vi "Custom User Scripting For New Override VI.vi"(8 "error in":errorcluster, 11 "VI Refnum in":refnum<vi>) -> (0 "error out":errorcluster)   [LabVIEW 2012]
doc: "When \"New >> VI For Override...\" is used to create a VI, this subVI will be invoked if the VI is created successfully after all other work to create the VI has been completed. Users may edit this subVI to add any instructions they wish for customizations of the newly generated VI."
uses:
  <vilib>/regexp/Match Regular Expression.xnode
  <vilib>/Utility/miscctls.llb/LVRectTypeDef.ctl
panel:
  out "error out 2":errorcluster
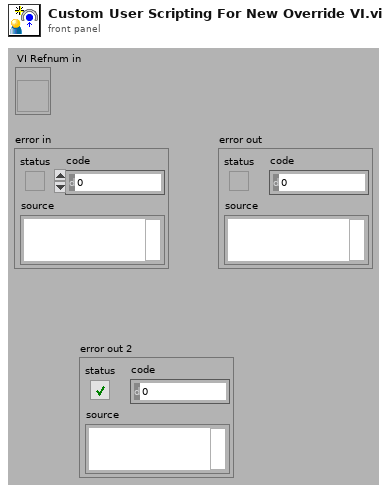
[diagram p1: front panel]
types:
  T1 = typedef "LVRectTypeDef.ctl" = cluster{"Left":i16, "Top":i16, "Right":i16, "Bottom":i16}
  T2 = cluster{"Class In":refnum<vi>, "Class Out":refnum<vi>, "Error In":refnum<vi>, "Error Out":refnum<vi>, "Other In":refnum<vi>[], "Other Out":refnum<vi>[]}
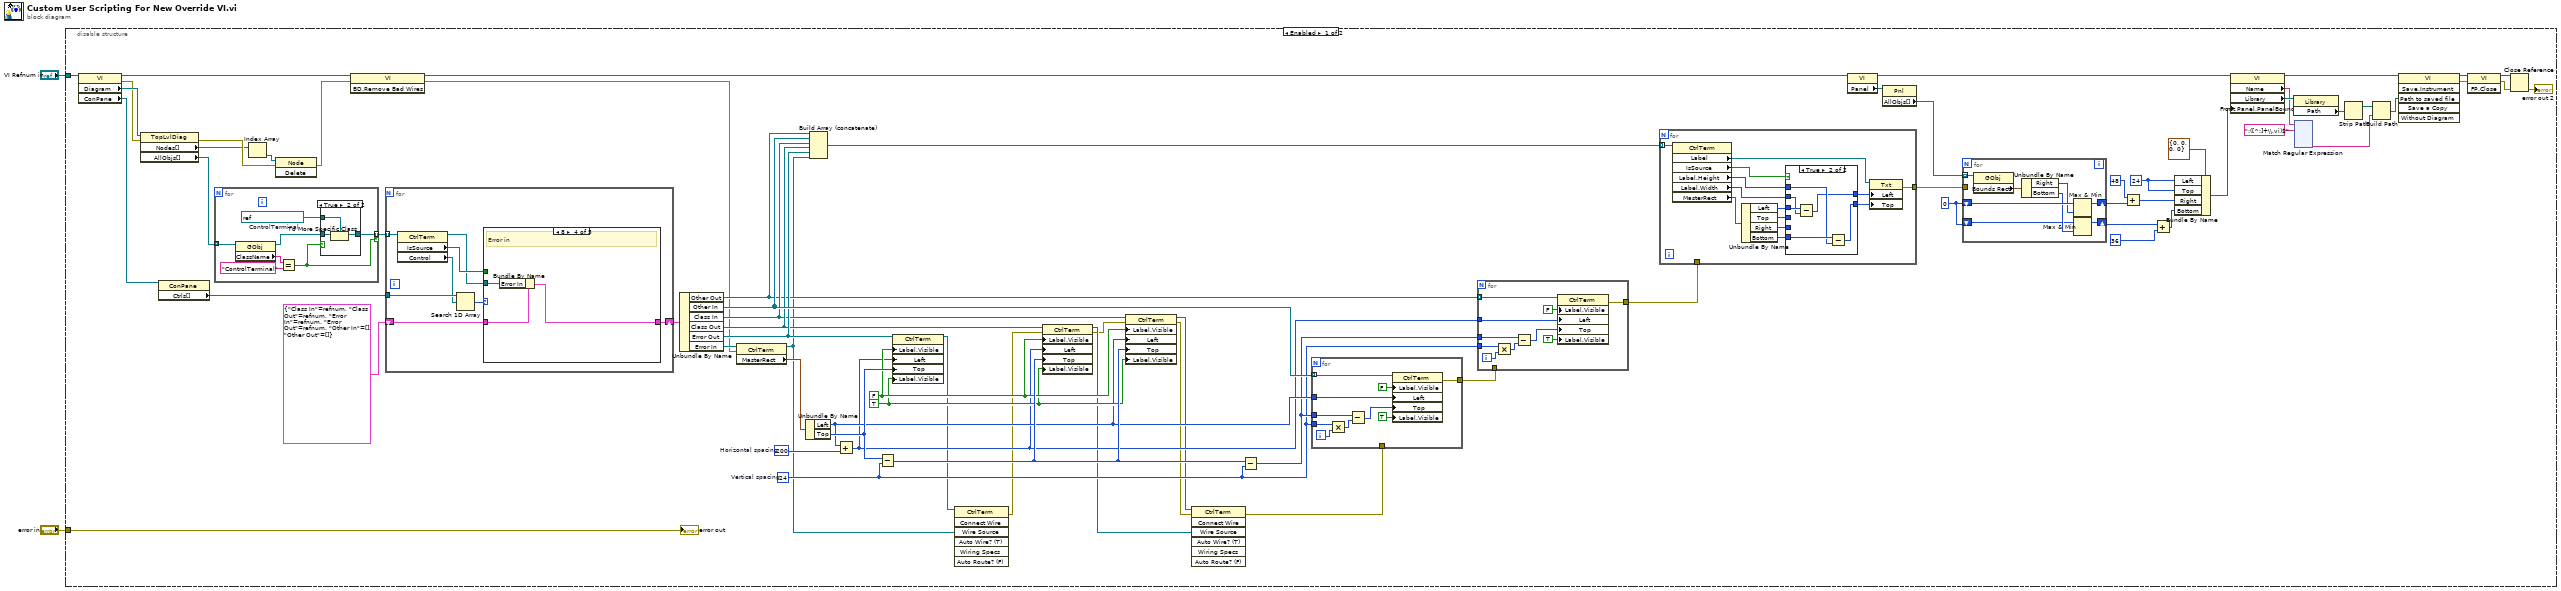
[diagram p0: block diagram]
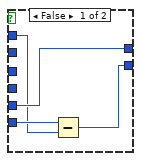
[diagram p2: hidden frame]
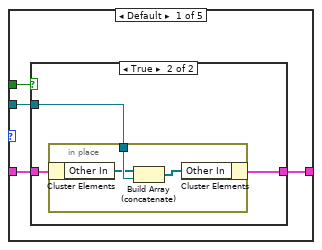
[diagram p3: hidden frame]
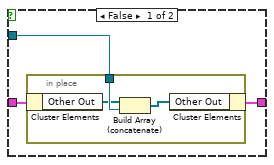
[diagram p4: hidden frame]
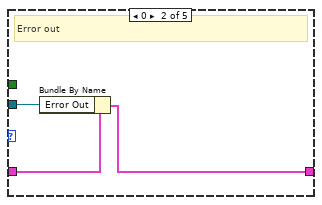
[diagram p5: hidden frame]
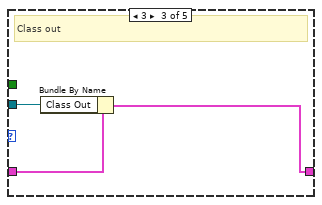
[diagram p6: hidden frame]
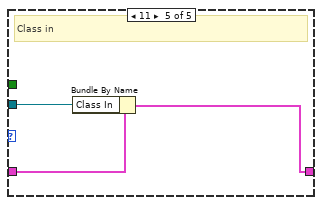
[diagram p7: hidden frame]
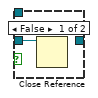
[diagram p8: hidden frame]
diagram:
  n1 = disable-structure shown="Enabled" {
    disable-tunnel: "error in" -> [w71 _]
    disable-tunnel: "VI Refnum in" -> [w70 _]
    frame Enabled {
      w13 = i16 24 ("x")
      w21 = i16 0 ("Right")
      w50 = TRUE ("Label.Visible")
      w51 = FALSE ("Label.Visible")
      w45 = 24  # Vertical spacing
      w61 = 200  # Horizontal spacing
      n2 = property class="VI"(reference=w70) -> (reference out=w24:refnum<vi>, error out=w66:errorcluster, "Diagram"=w69:refnum<vi>, "ConPane"=w39:refnum<vi>)  [unwired: 1 in]
      n3 = property class="TopLvlDiag"(reference=w69, error in=w66) -> (error out=w72:errorcluster, "Nodes[]"=w68:refnum<vi>[], "AllObjs[]"=w40:refnum<vi>[])  [unwired: 1 out]
      n4 = property class="ConPane"(reference=w39) -> ("Ctrls[]"=w64:refnum<vi>[])  [unwired: 1 in, 2 out]
      n5 = for {
        tunnel: w40 -> [w156] mode=indexing
        tunnel: [w151] -> w65 mode=indexing if=w150
        w152 = refnum<vi> refnum  # ControlTerminal
        n6 = property class="GObj"(reference=w156) -> (reference out=w153:refnum<vi>, "ClassName"=w155:string)  [unwired: 1 in, 1 out]
        n7 = Equal?(x=w155, y="ControlTerminal") -> (x = y?=w150:bool)
        n8 = case shown="True" w150 {
          tunnel: w153 -> [w157 w160]
          tunnel: w152 -> [_ w159]
          tunnel: [_ w158] -> w151
          frame False {
            n9 = Close Reference(reference=w157) -> ()  [unwired: 1 in, 1 out]
          }
          frame True {
            n10 = To More Specific Class(target class=w159, reference=w160) -> (specific class reference=w158:refnum<vi>)  [unwired: 1 in, 1 out]
          }
        }
      }
      n11 = Index Array(array=w68) -> (element=w67:refnum<vi>)  [unwired: 1 in]
      n12 = invoke class="Node" method="Delete"(reference=w67, error in=w72) -> (error out=w8:errorcluster)  [unwired: 1 in, 2 out]
      n13 = invoke class="VI" method="BD.Remove Bad Wires"(reference=w24, error in=w8) -> (reference out=w9:refnum<vi>, error out=w7:errorcluster)  [unwired: 1 in, 1 out]
      n14 = for {
        tunnel: w65 -> [w121] mode=indexing
        tunnel: w64 -> [w120]
        shift-right: [w115] -> w62
        shift-left: T2 {"Class In"=refnum, "Class Out"=refnum, "Error In"=refnum, "Error Out"=refnum, "Other In"=[], "Other Out"=[]} -> [w118]
        n15 = property class="CtrlTerm"(reference=w121) -> (reference out=w114:refnum<vi>, "IsSource"=w116:bool, "Control"=w117:refnum<vi>)  [unwired: 1 in, 1 out]
        n16 = Search 1D Array(1D array=w120, element=w117) -> (index of element=w119:i32)  [unwired: 1 in]
        n17 = case shown="8" w119 {
          tunnel: w118 -> [w124 w140 w143 w146 w149]
          tunnel: w114 -> [w123 w139 w142 w145 w148]
          tunnel: w116 -> [w125 _ _ _ _]
          tunnel: [w122 w138 w141 w144 w147] -> w115
          frame Default {
            n18 = case shown="True" w125 {
              tunnel: w124 -> [w128 w133]
              tunnel: w123 -> [w127 w134]
              tunnel: [w126 w132] -> w122
              frame False {
                n19 = in-place {
                  in-place-border: w127 -> [w131]
                  n20 = in-place-cluster #1(w128) -> ("Other Out"=w130:refnum<vi>[])
                  n21 = Build Array (concatenate)(w130, w131) -> (w129:refnum<vi>[])
                  n22 = in-place-cluster #1("Other Out"=w129) -> (w126:T2)
                }
              }
              frame True {
                n23 = in-place {
                  in-place-border: w134 -> [w137]
                  n24 = in-place-cluster #2(w133) -> ("Other In"=w136:refnum<vi>[])
                  n25 = Build Array (concatenate)(w136, w137) -> (w135:refnum<vi>[])
                  n26 = in-place-cluster #2("Other In"=w135) -> (w132:T2)
                }
              }
            }
          }
          frame 0 {
            # "Error out"
            n27 = Bundle By Name(cluster=w140, "Error Out"=w139) -> (w138:T2)
          }
          frame 3 {
            # "Class out"
            n28 = Bundle By Name(cluster=w143, "Class Out"=w142) -> (w141:T2)
          }
          frame 8 {
            # "Error in"
            n29 = Bundle By Name(cluster=w146, "Error In"=w145) -> (w144:T2)
          }
          frame 11 {
            # "Class in"
            n30 = Bundle By Name(cluster=w149, "Class In"=w148) -> (w147:T2)
          }
        }
      }
      n31 = Unbundle By Name(w62) -> ("Other Out"=w48:refnum<vi>[], "Other In"=w60:refnum<vi>[], "Class In"=w53:refnum<vi>, "Class Out"=w54:refnum<vi>, "Error Out"=w56:refnum<vi>, "Error In"=w58:refnum<vi>)
      n32 = property class="CtrlTerm"(reference=w58, error in=w7) -> (reference out=w44:refnum<vi>, "MasterRect"=w57:T1)  [unwired: 1 out]
      n33 = Unbundle By Name(w57) -> ("Left"=w49:i16, "Top"=w55:i16)
      n34 = Build Array (concatenate)(w48, w60, w53, w54, w56, w44) -> (w59:refnum<vi>[])
      n35 = Add(x=w49, y=w61) -> (x+y=w47:i32)
      n36 = Subtract(x=w55, y=w45) -> (x-y=w52:i32)
      n37 = property class="CtrlTerm"(reference=w56, "Label.Visible"=w51, "Left"=w47, "Top"=w55, "Label.Visible"=w50) -> (reference out=w43:refnum<vi>)  [unwired: 1 in, 1 out]
      n38 = invoke class="CtrlTerm" method="Connect Wire"(reference=w43, "Wire Source"=w44) -> (error out=w38:errorcluster)  [unwired: 5 in, 6 out]
      n39 = property class="CtrlTerm"(reference=w54, error in=w38, "Label.Visible"=w51, "Left"=w47, "Top"=w52, "Label.Visible"=w50) -> (reference out=w41:refnum<vi>, error out=w37:errorcluster)
      n40 = property class="CtrlTerm"(reference=w53, error in=w37, "Label.Visible"=w51, "Left"=w49, "Top"=w52, "Label.Visible"=w50) -> (reference out=w42:refnum<vi>, error out=w36:errorcluster)
      n41 = invoke class="CtrlTerm" method="Connect Wire"(reference=w42, error in=w36, "Wire Source"=w41) -> (error out=w35:errorcluster)  [unwired: 4 in, 6 out]
      n42 = Subtract(x=w52, y=w45) -> (x-y=w46:i32)
      n43 = for {
        tunnel: w45 -> [w170]
        tunnel: w46 -> [w168]
        tunnel: w60 -> [w166] mode=indexing
        tunnel: w49 -> [w163]
        tunnel: w35 -> [_]
        tunnel: [w161] -> w34
        i -> [w169]
        n44 = Multiply(x=w170, y=w169) -> (x*y=w167:i32)
        n45 = Subtract(x=w168, y=w167) -> (x-y=w165:i32)
        n46 = property class="CtrlTerm"(reference=w166, "Label.Visible"=FALSE, "Left"=w163, "Top"=w165, "Label.Visible"=TRUE) -> (error out=w161:errorcluster)  [unwired: 1 in, 1 out]
      }
      n47 = for {
        tunnel: w45 -> [w90]
        tunnel: w46 -> [w88]
        tunnel: w48 -> [w86] mode=indexing
        tunnel: w47 -> [w83]
        tunnel: w34 -> [_]
        tunnel: [w81] -> w33
        i -> [w89]
        n48 = Multiply(x=w90, y=w89) -> (x*y=w87:i32)
        n49 = Subtract(x=w88, y=w87) -> (x-y=w85:i32)
        n50 = property class="CtrlTerm"(reference=w86, "Label.Visible"=FALSE, "Left"=w83, "Top"=w85, "Label.Visible"=TRUE) -> (error out=w81:errorcluster)  [unwired: 1 in, 1 out]
      }
      n51 = for {
        tunnel: w59 -> [w103] mode=indexing
        tunnel: w33 -> [_]
        tunnel: [w91] -> w23
        n52 = property class="CtrlTerm"(reference=w103) -> ("Label"=w102:refnum<vi>, "IsSource"=w100:bool, "Label.Height"=w99:u32, "Label.Width"=w98:u32, "MasterRect"=w101:T1)  [unwired: 1 in, 2 out]
        n53 = Unbundle By Name(w101) -> ("Left"=w97:i16, "Top"=w96:i16, "Right"=w95:i16, "Bottom"=w94:i16)
        n54 = case shown="True" w100 {
          tunnel: w99 -> [w105 w112]
          tunnel: w98 -> [_ w110]
          tunnel: w97 -> [_ w111]
          tunnel: w96 -> [_ _]
          tunnel: w95 -> [w107 _]
          tunnel: w94 -> [w106 w113]
          tunnel: [w107 w108] -> w93
          tunnel: [w104 w109] -> w92
          frame False {
            n55 = Subtract(x=w106, y=w105) -> (x-y=w104:u32)
          }
          frame True {
            n56 = Subtract(x=w111, y=w110) -> (x-y=w108:u32)
            n57 = Subtract(x=w113, y=w112) -> (x-y=w109:u32)
          }
        }
        n58 = property class="Txt"(reference=w102, "Left"=w93, "Top"=w92) -> (error out=w91:errorcluster)  [unwired: 1 in, 1 out]
      }
      n59 = property class="VI"(reference=w9) -> (reference out=w14:refnum<vi>, "Panel"=w25:refnum<vi>)  [unwired: 1 in, 1 out]
      n60 = property class="Pnl"(reference=w25) -> ("AllObjs[]"=w22:refnum<vi>[])  [unwired: 1 in, 2 out]
      n61 = for {
        tunnel: w23 -> [_]
        tunnel: w22 -> [w80] mode=indexing
        shift-right: [w77] -> w17
        shift-left: w21 -> [w78]
        shift-right: [w76] -> w18
        shift-left: w21 -> [w73]
        n62 = property class="GObj"(reference=w80) -> ("Bounds Rect"=w79:T1)  [unwired: 1 in, 2 out]
        n63 = Unbundle By Name(w79) -> ("Right"=w75:i16, "Bottom"=w74:i16)
        n64 = Max & Min(x=w78, y=w75) -> (max(x,y)=w77:i16)  [unwired: 1 out]
        n65 = Max & Min(x=w73, y=w74) -> (max(x,y)=w76:i16)  [unwired: 1 out]
      }
      n66 = Add(x=i16 48, y=w17) -> (x+y=w16:i16)
      n67 = Add(x=w18, y=i16 36 ("x")) -> (x+y=w15:i16)
      n68 = Bundle By Name(cluster=T1 {"Left"=0, "Top"=0, "Right"=0, "Bottom"=0} ("Front Panel Window:Panel Bounds"), "Left"=w13, "Top"=w13, "Right"=w16, "Bottom"=w15) -> (w19:T1)
      n69 = property class="VI"(reference=w14, "Front Panel.PanelBounds"=w19) -> ("Name"=w28:string, "Library"=w32:refnum<vi>)  [unwired: 1 in, 2 out]
      n70 = property class="Library"(reference=w32) -> ("Path"=w31:path)  [unwired: 1 in, 2 out]
      n71 = xnode "Match Regular Expression"("input string"=w28, "regular expression"=":([^:]+\\.vi)$") -> ("submatch 1"=w26:string)  [unwired: 4 in, 5 out]
      n72 = Strip Path(path=w31) -> (stripped path=w30:path)  [unwired: 1 out]
      n73 = Build Path(base path=w30, name or relative path=w26) -> (appended path=w29:path)
      n74 = invoke class="VI" method="Save.Instrument"(reference=w14, "Path to saved file"=w29) -> (reference out=w10:refnum<vi>, error out=w4:errorcluster)  [unwired: 4 in, 4 out]
      n75 = invoke class="VI" method="FP.Close"(reference=w10, error in=w4) -> (reference out=w6:refnum<vi>, error out=w5:errorcluster)  [unwired: 1 in, 1 out]
      n76 = Close Reference(reference=w6, error in (no error)=w5) -> (error out=→"error out 2":errorcluster)
      "error out" <- w71
    }
    frame Disabled {
    }
  }
